vi "json approval test.vi"   [LabVIEW 2020]
uses:
  Common/Person/Person.lvclass
  Common/Person/Person.lvclass/Person.ctl
  <vilib>/addons/_JKI Toolkits/Caraya/classes/Test/Test.lvclass
  <vilib>/SAS/Approval Tests/Extensions/Caraya.Extension/lib_Caraya.Extension.lvlib
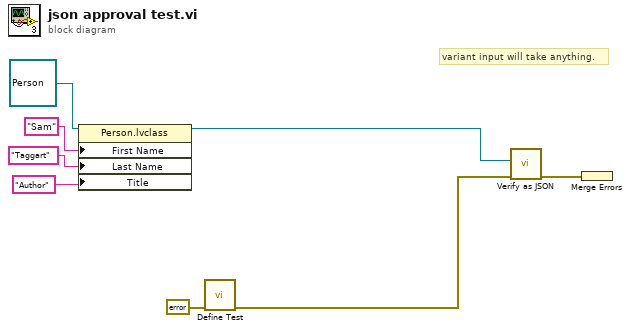
[diagram p0: block diagram]
diagram:
  # "variant input will take anything."
  n1 = property on="Property Node" class="Person.lvclass"(reference=refnum<class "Person.lvclass"> refnum ("Person.lvclass"), "First Name"="Sam" ("Test Data"), "Last Name"="Taggart" ("Test Data"), "Title"="Author" ("Test Data")) -> (reference out=w1:refnum<class "Person.lvclass">)  [unwired: 1 in, 1 out]
  n2 = call <vilib>:"Define Test.vi"("error in (no error)"=errorcluster {"status"=FALSE, "code"=0, "source"=""}) -> ("error out"=w2:errorcluster)  [unwired: 9 in, 1 out]
  n3 = call <vilib>:"Verify as JSON.vi"("error in"=w2, "Anything"=w1) -> ("error out"=w3:errorcluster)  [unwired: 8 in, 1 out]
  n4 = Merge Errors(w3) -> ()  [unwired: 1 out]
